vi "OAT Polar Plot (Auto Label).vi"(0 "picture":picture, 1 "picture\ndimensions (w,h)":cluster{"width":u32, "height":u32}, 2 "polar settings":T3={"polar attributes"={"maximum"=0.0, "minimum"=0.0, "clip to min"=FALSE, "log"=FALSE, "grid color"=3381657, "plot color"=16711680, "fmt and prec"={"format"=enum."Scientific", "precision"=1}, "visible section"=8}, "desired font(Application)"=enum."Application Font", "[user-specified font]"={"Font Name"="", "Size"=0, "Strikeout?"=FALSE, "Italic?"=FALSE, "Underline?"=FALSE, "Outline?"=FALSE, "Shadow?"=FALSE, "Bold?"=FALSE}} {"polar attributes"."minimum" format="%.2f"; "polar attributes"."maximum" format="%.2f"}, 3 "cursor attributes":T4={"layout color"=852223, "active color"=16740820, "precision"=2, "BG transparent? (T)"=TRUE, "radius"=2}, 5 "magnitude":cluster{"time/rev/rpm":dbl[], "magnitude":dbl[]} {"magnitude" format="%.2f"; "time/rev/rpm" format="%.2f"}, 7 "phase [phase lag]":cluster{"time/rev/rpm":dbl[], "phase":dbl[]} {"phase" format="%.2f"; "time/rev/rpm" format="%.2f"}, 11 "error in (no error)":errorcluster, 12 "channel settings":T2 {"probe angle [deg]" max=360 step=1; "shaft rotating direction" items=["CCW", "CW"]}, 13 "view info":T1={"dB on? (F)"=FALSE, "unwrap phase? (T)"=TRUE, "unit in degree? (T)"=TRUE}, 14 "avoid overlap? (T)":bool=TRUE) -> (4 "new picture":picture, 15 "error out":errorcluster)   [LabVIEW 2017]
doc: "Draws a polar plot on a picture control and adds labels. The polar plot displays the magnitude and phase of a certain order on a picture control. You must manually select the polymorphic instance to use. Use the Manual Label instance if you want to label the polar plot manually."
uses:
  <vilib>/addons/Sound and Vibration/Order Analysis/Backward Compatibility/SubVIs/OAT Polar Cursor Attributes.ctl
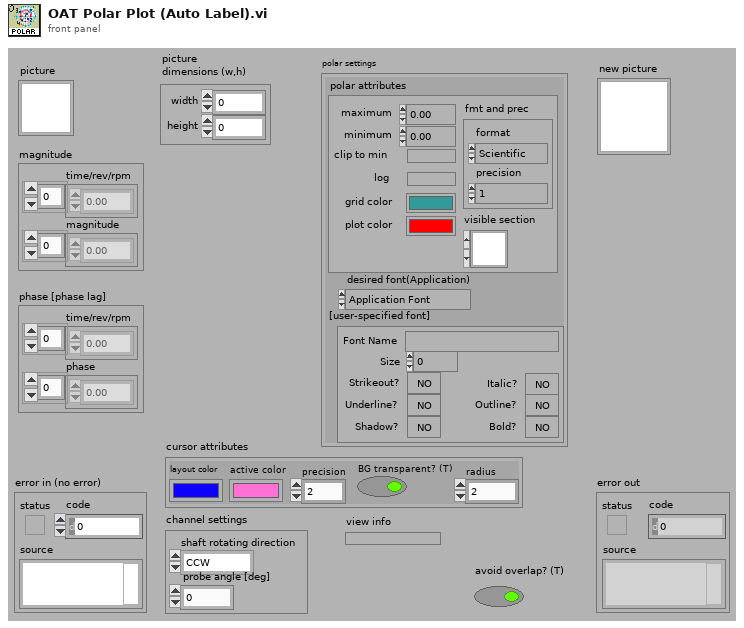
[diagram p1: front panel]
types:
  T1 = cluster{"dB on? (F)":bool, "unwrap phase? (T)":bool, "unit in degree? (T)":bool}
  T2 = cluster{"shaft rotating direction":u16, "probe angle [deg]":u16}
  T3 = cluster{"polar attributes":cluster{"maximum":dbl, "minimum":dbl, "clip to min":bool, "log":bool, "grid color":u32, "plot color":u32, "fmt and prec":cluster{"format":enum8{"Decimal", "Scientific", "Engineering", "Binary", "Octal", "Hex"}, "precision":u8}, "visible section":u16}, "desired font(Application)":enum16{"User-specified Font", "Application Font", "System Font", "Dialog Font"}, "[user-specified font]":cluster{"Font Name":string, "Size":i16, "Strikeout?":bool, "Italic?":bool, "Underline?":bool, "Outline?":bool, "Shadow?":bool, "Bold?":bool}}
  T4 = typedef "OAT Polar Cursor Attributes.ctl" = cluster{"layout color":u32, "active color":u32, "precision":i16, "BG transparent? (T)":bool, "radius":i16}
  T5 = cluster{"maximum":dbl, "minimum":dbl, "clip to min":bool, "log":bool, "grid color":u32, "plot color":u32, "fmt and prec":cluster{"format":enum8{"Decimal", "Scientific", "Engineering", "Binary", "Octal", "Hex"}, "precision":u8}, "visible section":u16}
  T6 = cluster{"Name":string, "Location":cluster{"mag":dbl, "phase":dbl}}[]
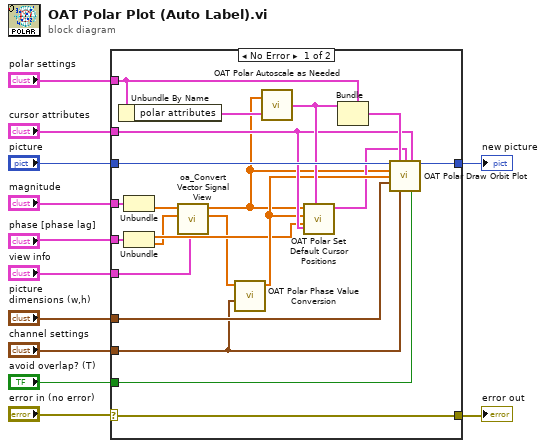
[diagram p0: block diagram]
diagram:
  n1 = case shown="No Error" "error in (no error)" {
    selector: "error in (no error)" -> [w20 w35]
    tunnel: "polar settings" -> [w33 _]
    tunnel: [w32 w34] -> w11
    tunnel: "magnitude" -> [w31 _]
    tunnel: "phase [phase lag]" -> [w30 _]
    tunnel: "avoid overlap? (T)" -> [w29 _]
    tunnel: "picture" -> [w26 w34]
    tunnel: "cursor attributes" -> [w24 _]
    tunnel: "picture\ndimensions (w,h)" -> [w23 _]
    tunnel: "view info" -> [w14 _]
    tunnel: "channel settings" -> [w13 _]
    tunnel: [w20 w35] -> w1
    frame No Error {
      n2 = Unbundle By Name(w33) -> ("polar attributes"=w27:T5)
      n3 = Unbundle(w31) -> ("magnitude"=w17:dbl[])  [unwired: 1 out]
      n4 = Unbundle(w30) -> ("time/rev/rpm"=w19:dbl[], "phase"=w15:dbl[])
      n5 = call <vilib>:"oa_Convert Vector Signal View.vi"("view"=w14, "phase"=w15, "magnitude"=w17) -> ("phase out"=w18:dbl[], "magnitude out"=w16:dbl[])  [unwired: 7 in]
      n6 = call <vilib>:"OAT Polar Phase Value Conversion.vi"("channel settings"=w13, "phases in"=w18) -> ("phases out"=w22:dbl[])  [unwired: 9 in]
      n7 = call <vilib>:"OAT Polar Autoscale as Needed.vi"("polar attributes"=w27, "magnitudes (even angular)"=w16) -> ("polar attributes"=w25:T5)
      n8 = call <vilib>:"OAT Polar Set Default Cursor Positions.vi"("cursor attributes"=w24, "polar attributes"=w25, "cursor values"=w19, "phases"=w22, "magnitudes (even angular)"=w16) -> ("Cursor List (EU position]"=w21:T6)  [unwired: 6 in]
      n9 = Bundle(cluster=w33, "polar attributes"=w25) -> (w28:T3)  [unwired: 2 in]
      n10 = call <vilib>:"OAT Polar Draw Orbit Plot.vi"("picture"=w26, "polar settings"=w28, "Cursor List (EU position]"=w21, "cursor attributes"=w24, "magnitudes (even angular)"=w16, "phases"=w22, "picture \ndimensions (w,h)"=w23, "channel settings"=w13, "avoid overlap? (Y)"=w29) -> ("picture out"=w32:picture)  [unwired: 5 in, 1 out]
    }
    frame Error {
    }
  }
  "new picture" <- w11
  "error out" <- w1
